vi "Split.vi"(7 "Round up?":bool, 8 "Val":u64, 9 "Label":string, 10 "Cluster":T1) -> (2 "Result":T1[](array[typedef]))   [LabVIEW 2021, in "Rule.lvclass"]
uses:
  Rule.lvclass
  xmas.ctl
  Rule.lvclass/Rule.ctl
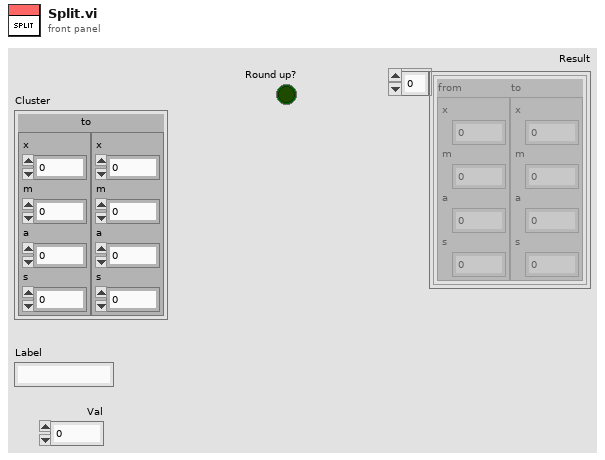
[diagram p1: front panel]
types:
  T1 = typedef "xmas.ctl" = cluster{"from":cluster{"x":u64, "m":u64, "a":u64, "s":u64}, "to":cluster{"x":u64, "m":u64, "a":u64, "s":u64}}
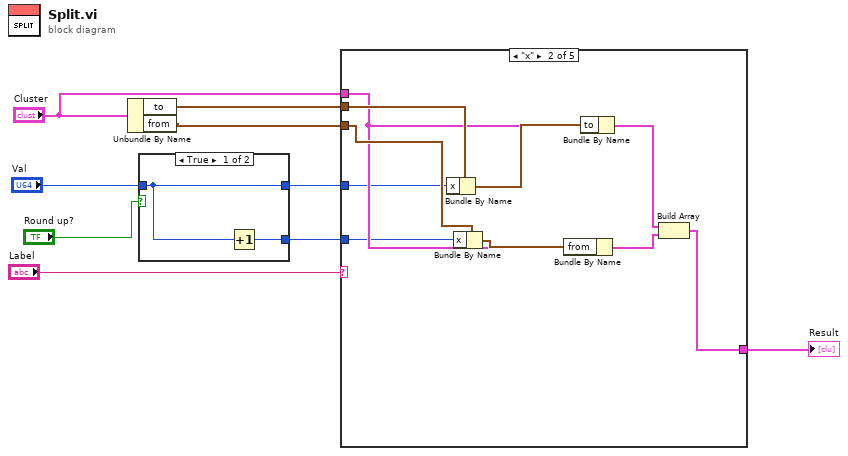
[diagram p0: block diagram]
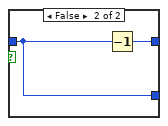
[diagram p2: hidden frame]
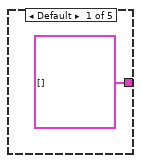
[diagram p3: hidden frame]
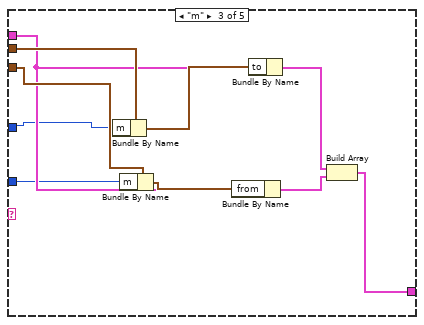
[diagram p4: hidden frame]
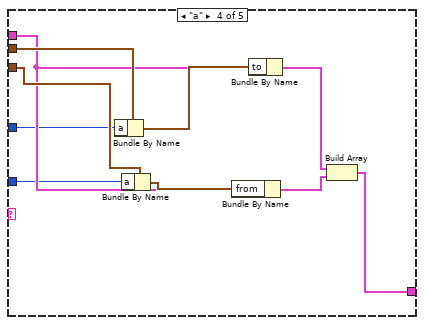
[diagram p5: hidden frame]
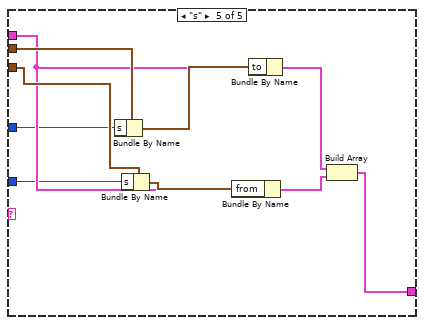
[diagram p6: hidden frame]
diagram:
  n1 = Unbundle By Name("Cluster") -> ("to"=w8:cluster{"x":u64, "m":u64, "a":u64, "s":u64}, "from"=w7:cluster{"x":u64, "m":u64, "a":u64, "s":u64})
  n2 = case shown="True" "Round up?" {
    tunnel: "Val" -> [w11 w13]
    tunnel: [w11 w12] -> w2
    tunnel: [w10 w13] -> w1
    frame True {
      n3 = Increment(x=w11) -> (x+1=w10:u64)
    }
    frame False {
      n4 = Decrement(x=w13) -> (x-1=w12:u64)
    }
  }
  n5 = case shown="\"x\"" "Label" {
    tunnel: w8 -> [_ w21 w31 w41 w51]
    tunnel: w7 -> [_ w23 w33 w43 w53]
    tunnel: "Cluster" -> [_ w18 w28 w38 w48]
    tunnel: [T1[] [] w17 w27 w37 w47] -> w4
    tunnel: w2 -> [_ w16 w26 w36 w46]
    tunnel: w1 -> [_ w15 w25 w35 w45]
    frame Default {
    }
    frame "x" {
      n6 = Bundle By Name(cluster=w21, "x"=w16) -> (w24:cluster{"x":u64, "m":u64, "a":u64, "s":u64})
      n7 = Bundle By Name(cluster=w23, "x"=w15) -> (w22:cluster{"x":u64, "m":u64, "a":u64, "s":u64})
      n8 = Bundle By Name(cluster=w18, "from"=w22) -> (w19:T1)
      n9 = Bundle By Name(cluster=w18, "to"=w24) -> (w20:T1)
      n10 = Build Array(w20, w19) -> (w17:T1[])
    }
    frame "m" {
      n11 = Bundle By Name(cluster=w31, "m"=w26) -> (w34:cluster{"x":u64, "m":u64, "a":u64, "s":u64})
      n12 = Bundle By Name(cluster=w33, "m"=w25) -> (w32:cluster{"x":u64, "m":u64, "a":u64, "s":u64})
      n13 = Bundle By Name(cluster=w28, "from"=w32) -> (w29:T1)
      n14 = Bundle By Name(cluster=w28, "to"=w34) -> (w30:T1)
      n15 = Build Array(w30, w29) -> (w27:T1[])
    }
    frame "a" {
      n16 = Bundle By Name(cluster=w41, "a"=w36) -> (w44:cluster{"x":u64, "m":u64, "a":u64, "s":u64})
      n17 = Bundle By Name(cluster=w43, "a"=w35) -> (w42:cluster{"x":u64, "m":u64, "a":u64, "s":u64})
      n18 = Bundle By Name(cluster=w38, "from"=w42) -> (w39:T1)
      n19 = Bundle By Name(cluster=w38, "to"=w44) -> (w40:T1)
      n20 = Build Array(w40, w39) -> (w37:T1[])
    }
    frame "s" {
      n21 = Bundle By Name(cluster=w51, "s"=w46) -> (w54:cluster{"x":u64, "m":u64, "a":u64, "s":u64})
      n22 = Bundle By Name(cluster=w53, "s"=w45) -> (w52:cluster{"x":u64, "m":u64, "a":u64, "s":u64})
      n23 = Bundle By Name(cluster=w48, "from"=w52) -> (w49:T1)
      n24 = Bundle By Name(cluster=w48, "to"=w54) -> (w50:T1)
      n25 = Build Array(w50, w49) -> (w47:T1[])
    }
  }
  "Result" <- w4
